vi "Record data.vi"(7 "File":path=path "C:/ni-rt/Record 3.xml") -> ()   [LabVIEW 2012]
uses:
  <vilib>/Rock Robotics/SystemInterfaces/DIO/FPGA_DIOPWMChannel.ctl
  <vilib>/Rock Robotics/WPI/MotorControl/WPI_MotorControlOpen Talon.vi
  <vilib>/Rock Robotics/WPI/Joystick/WPI_JoystickGetSetRefNum.vi
  <vilib>/Rock Robotics/WPI/Solenoid/WPI_SolenoidGetEnum.vi
panel:
  in  "Start Loop":bool
  in  "Stop Loop":bool
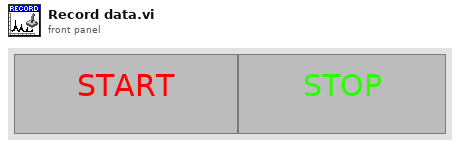
[diagram p1: front panel]
types:
  T1 = typedef "FPGA_DIOPWMChannel.ctl" = enum8{"PWM 1", "PWM 2", "PWM 3", "PWM 4", "PWM 5", "PWM 6", "PWM 7", "PWM 8", "PWM 9", "PWM 10", "Invalid"}
  T2 = typedef "WPI_MotorControlDeviceRef.ctl" = cluster{"DeviceStatus":errorcluster, "Type":enum16{"PWM", "CAN"}, "PWM":cluster{"Digital Module":T3, "PWM Channel":T1, "DeadBand":T4}, "CAN":cluster{"Device Number":u8, "Control Mode":T5, "Semaphore":T6, "Max Vout":dbl}, "Invert":bool, "TransformRef":T7, "InvTransformRef":T7}
  T3 = typedef "FPGA_TypedefDigitalModule.ctl" = enum16{"Digital Module 1", "Digital Module 2"}
  T4 = typedef "WPI_PWMDeadband.ctl" = cluster{"Name":string, "maxPositivePwm":i32, "minPositivePwm":i32, "centerPwm":i32, "maxNegativePwm":i32, "minNegativePwm":i32, "angularRange":u16}
  T5 = typedef "WPI_CANJaguar_ControlMode.ctl" = enum8{"Percent VBus", "Current", "Speed", "Position", "Voltage"}
  T6 = typedef "Semaphore RefNum" = refnum<k1>
  T7 = typedef "WPI_PWMTransform_ConPane.ctl" = refnum<vi>
  T8 = typedef "WPI_JoystickDevRef.ctl" = cluster{"Device":T9}
  T9 = typedef "WPI_JoystickDeviceEnum.ctl" = enum16{"USB 1", "USB 2", "USB 3", "USB 4", "Kinect 1", "Kinect 2"}
  T10 = typedef "WPI_SolenoidDevRef.ctl" = cluster{"DevStatus":errorcluster, "Solenoid Module":T11, "Forward Solenoid Channel":T12, "Reverse Solenoid Channel":T12}
  T11 = typedef "FPGA_TypedefSolenoidModule.ctl" = enum16{"Solenoid Module 1", "Solenoid Module 2"}
  T12 = typedef "WPI_SolenoidChannel.ctl" = enum8{"Solenoid 1", "Solenoid 2", "Solenoid 3", "Solenoid 4", "Solenoid 5", "Solenoid 6", "Solenoid 7", "Solenoid 8", "Invalid"}
  T13 = cluster{"axis 1 (x)":dbl, "axis 2 (y)":dbl, "axis 3 (throttle)":dbl, "axis 4":dbl, "axis 5":dbl, "axis 6":dbl}
  T14 = typedef "WPI_SolenoidValue.ctl" = enum16{"Off", "On", "Forward", "Reverse"}
  T15 = cluster{"Output":dbl, "Output":dbl, "axis 3 (throttle)":dbl, "Output":dbl, "Output":dbl, "Value":T14}
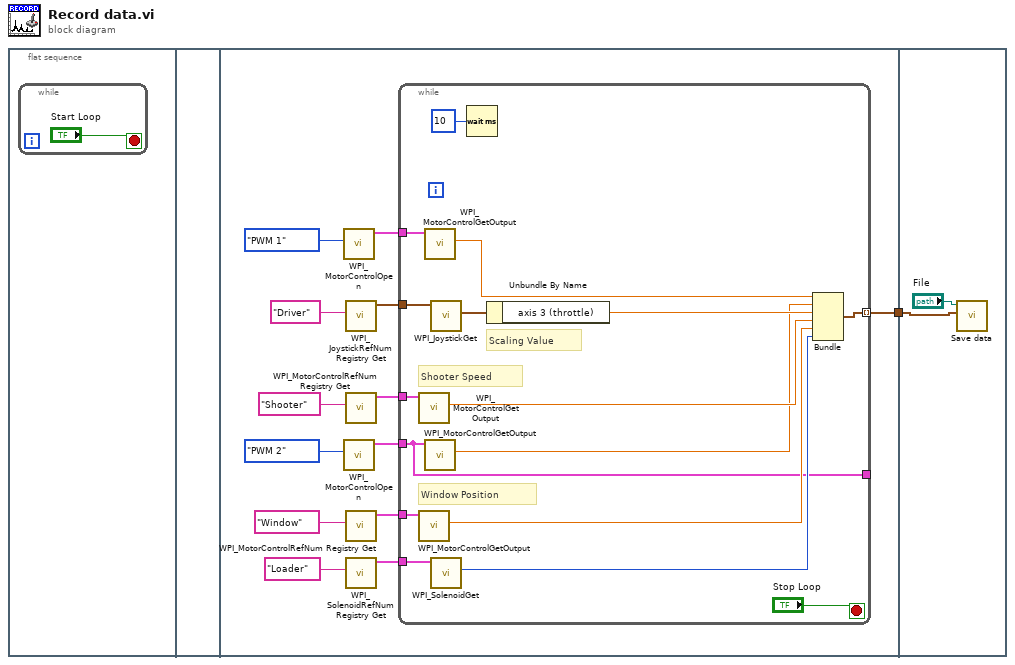
[diagram p0: block diagram]
diagram:
  n1 = flat-sequence {
    tunnel: [w15] -> w1
    tunnel: w1 -> [w32]
    frame #0 {
      n2 = while {
        stop <- "Start Loop" stop-if-true
      }
    }
    frame #1 {
    }
    frame #2 {
      n3 = call-poly <vilib>:"WPI_MotorControlOpen.vi"("PWM Channel"=FPGA_DIOPWMChannel."PWM 1") -> ("MotorControlDeviceRef"=w6:T2)  [unwired: 9 in, 1 out]
      n4 = call-poly <vilib>:"WPI_MotorControlOpen.vi"("PWM Channel"=FPGA_DIOPWMChannel."PWM 2") -> ("MotorControlDeviceRef"=w5:T2)  [unwired: 9 in, 1 out]
      n5 = call <vilib>:"WPI_JoystickRefNum Registry Get.vi"("refnum name"="Driver") -> ("JoystickDevRef"=w13:T8)  [unwired: 9 in, 1 out]
      n6 = call <vilib>:"WPI_MotorControlRefNum Registry Get.vi"("refnum name"="Shooter") -> ("MotorControlDevRef"=w7:T2)  [unwired: 9 in, 1 out]
      n7 = call <vilib>:"WPI_MotorControlRefNum Registry Get.vi"("refnum name"="Window") -> ("MotorControlDevRef"=w8:T2)  [unwired: 9 in, 1 out]
      n8 = call <vilib>:"WPI_SolenoidRefNum Registry Get.vi"("refnum name"="Loader") -> ("SolenoidDevRef"=w12:T10)  [unwired: 9 in, 1 out]
      n9 = while {
        tunnel: [w31] -> w15 mode=indexing
        tunnel: w13 -> [w23]
        tunnel: w12 -> [w22]
        tunnel: w8 -> [w21]
        tunnel: w7 -> [w20]
        tunnel: [w18] -> _
        tunnel: w6 -> [w19]
        tunnel: w5 -> [w18]
        stop <- "Stop Loop" stop-if-true
        # "Window Position"
        # "Shooter Speed"
        # "Scaling Value"
        n10 = call <vilib>:"WPI_MotorControlGetOutput.vi"("MotorControlDevRef"=w20) -> ("Output"=w26:dbl)  [unwired: 8 in, 2 out]
        n11 = call <vilib>:"WPI_MotorControlGetOutput.vi"("MotorControlDevRef"=w21) -> ("Output"=w25:dbl)  [unwired: 8 in, 2 out]
        n12 = call <vilib>:"WPI_MotorControlGetOutput.vi"("MotorControlDevRef"=w19) -> ("Output"=w16:dbl)  [unwired: 8 in, 2 out]
        n13 = call <vilib>:"WPI_MotorControlGetOutput.vi"("MotorControlDevRef"=w18) -> ("Output"=w17:dbl)  [unwired: 8 in, 2 out]
        n14 = call <vilib>:"WPI_JoystickGet.vi"("JoystickDevRef"=w23) -> ("Axes"=w28:T13)  [unwired: 4 in, 2 out]
        n15 = call-poly <vilib>:"WPI_SolenoidGet.vi"("SolenoidDevRef"=w22) -> ("Value"=w24:T14)  [unwired: 8 in, 2 out]
        n16 = Wait (ms)(milliseconds to wait=u32 10) -> ()  [unwired: 1 out]
        n17 = Unbundle By Name(w28) -> ("axis 3 (throttle)"=w27:dbl)
        n18 = Bundle("Output"=w16, "Output"=w17, "axis 3 (throttle)"=w27, "Output"=w26, "Output"=w25, "Value"=w24) -> (w31:T15)  [unwired: 1 in]
      }
    }
    frame #3 {
      n19 = call "Save data.vi"("Auto Data"=w32, "File"="File") -> ()  [unwired: 10 in]
    }
  }
